vi "test Set and Get All Log File Properties.vi"(8 "error in (no error)":errorcluster, 11 "TestCase in":refnum<class "Embedded Data Logger Scripting Unit Tests.lvclass">) -> (0 "error out":errorcluster, 3 "TestCase out":refnum<class "Embedded Data Logger Scripting Unit Tests.lvclass">)   [LabVIEW 2027, in "Embedded Data Logger Scripting Unit Tests.lvclass"]
uses:
  Embedded Data Logger Scripting Unit Tests.lvclass
  C:/Program Files/National Instruments/LabVIEW 2027/vi.lib/NI/VeriStand Custom Device Testing Tools/VeriStandScriptingTestCase/VeriStandScriptingTestCase.lvclass
  Shared/Segment Files By.ctl
  <vilib>/NI/VeriStand Custom Device Testing Tools/VeriStandScriptingTestCase/VeriStandScriptingTestCase.lvclass/VeriStandScriptingTestCase.ctl
  <vilib>/NI/VeriStand Custom Device Testing Tools/VeriStandScriptingTestCase/Read Target.vi
  C:/NetCoreDLL/NationalInstruments.VeriStand.SystemDefinitionAPI.dll
  NetCoreDLL/NationalInstruments.VeriStand.SystemDefinitionAPI.dll
  Embedded Data Logger Scripting.lvlib
  Shared/Embedded Data Logger Shared.lvlib
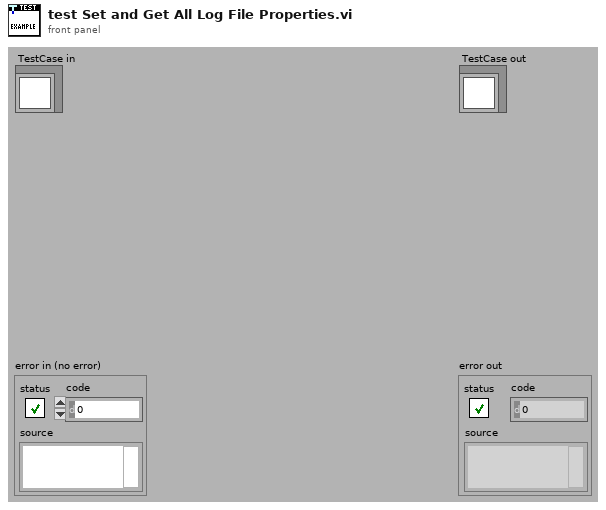
[diagram p1: front panel]
types:
  T1 = typedef "Embedded Data Logger Shared.lvlib/Segment Files By.ctl" = enum16{"Time", "Size"}
  T2 = typedef "Custom Device API.lvlib/Custom Device Item Ref.ctl" = u64
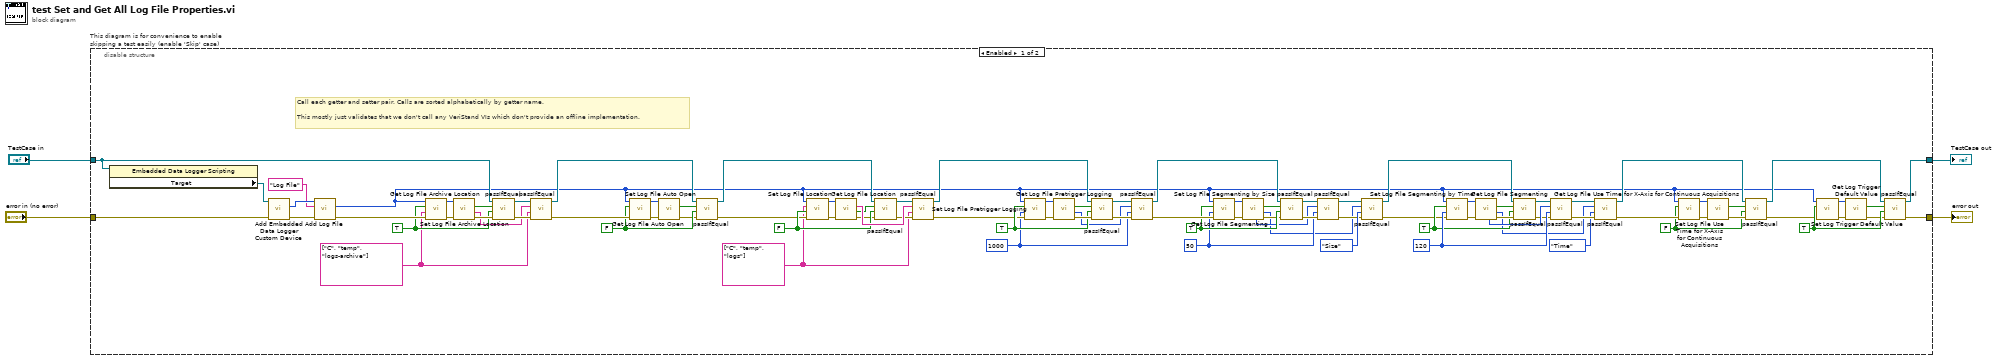
[diagram p0: block diagram]
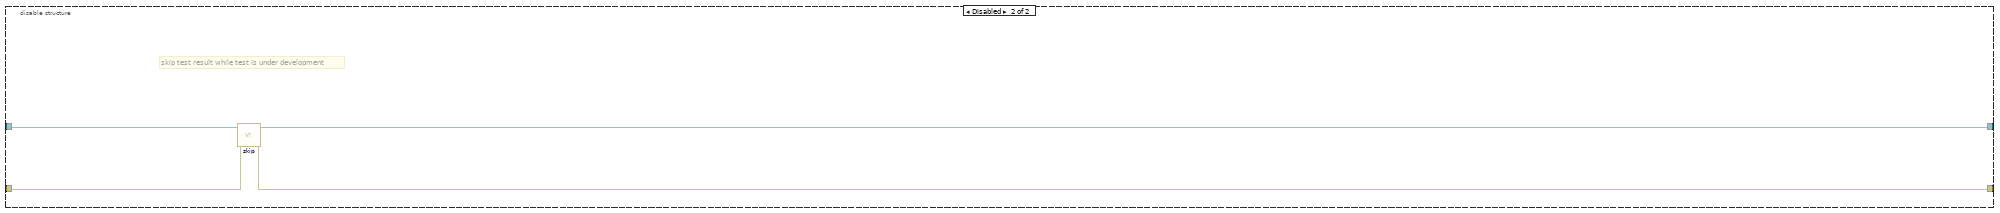
[diagram p2: hidden frame]
diagram:
  n1 = disable-structure "This diagram is for convenience to enable skipping a test easily (enable 'Skip' case)" shown="Enabled" {
    disable-tunnel: "TestCase in" -> [w86 w100]
    disable-tunnel: [w8 w98] -> w1
    disable-tunnel: [w9 w99] -> w3
    disable-tunnel: "error in (no error)" -> [w92 w97]
    frame Enabled {
      w14 = TRUE ("auto open")
      w15 = FALSE ("auto open")
      w33 = u32 120 ("file size (MB)")
      w29 = TRUE ("segment into multiple files")
      w42 = u32 50 ("file size (MB)")
      w47 = TRUE ("segment into multiple files")
      w52 = 1000 ("pretrigger samples")
      w62 = TRUE ("auto open")
      w64 = string[] ["C", "temp", "logs"] ("archive directory parts")
      w71 = FALSE ("archive closed log files")
      w76 = FALSE ("auto open")
      w83 = string[] ["C", "temp", "logs-archive"] ("archive directory parts")
      w84 = TRUE ("archive closed log files")
      # "Call each getter and setter pair. Calls are sorted alphabetically by getter name. \n\nThis mostly just validates that we don't call any VeriStand VIs which don't provide an offline implementation."
      n2 = property class="Embedded Data Logger Scripting "(reference=w86) -> ("Target"=w93:refnum<k39>)  [unwired: 1 in, 2 out]
      n3 = call "Add Embedded Data Logger Custom Device.vi"("error in"=w92, "NationalInstruments.VeriStand.SystemDefinitionAPI.Target"=w93) -> ("error out"=w95:errorcluster, "embedded data logger"=w96:T2)  [unwired: 7 in, 1 out]
      n4 = call "Add Log File.vi"("error in"=w95, "log file name"="Log File", "embedded data logger in"=w96) -> ("error out"=w89:errorcluster, "log file"=w5:T2)  [unwired: 6 in, 1 out]
      n5 = call "Set Log File Archive Location.vi"("error in (no error)"=w89, "archive directory parts"=w83, "archive closed log files"=w84, "log file in"=w5) -> ("error out"=w91:errorcluster, "log file out"=w90:T2)  [unwired: 6 in]
      n6 = call "Get Log File Archive Location.vi"("error in (no error)"=w91, "log file in"=w90) -> ("error out"=w88:errorcluster, "archive directory parts"=w82:string[], "archive closed log files"=w85:bool)  [unwired: 6 in, 1 out]
      n7 = call-dynamic "passIfEqual.vi"("error in (no error)"=w88, "y"=w84, "x"=w85, "TestCase in"=w86) -> ("error out"=w87:errorcluster, "TestCase out"=w81:refnum<class "Embedded Data Logger Scripting Unit Tests.lvclass">)  [unwired: 6 in]
      n8 = call-dynamic "passIfEqual.vi"("error in (no error)"=w87, "y"=w83, "x"=w82, "TestCase in"=w81) -> ("error out"=w80:errorcluster, "TestCase out"=w74:refnum<class "Embedded Data Logger Scripting Unit Tests.lvclass">)  [unwired: 6 in]
      n9 = call "Set Log File Auto Open.vi"("error in"=w80, "auto open"=w76, "log file in"=w5) -> ("error out"=w78:errorcluster, "log file out"=w79:T2)  [unwired: 7 in]
      n10 = call "Get Log File Auto Open.vi"("error in"=w78, "log file in"=w79) -> ("error out"=w75:errorcluster, "auto open"=w77:bool)  [unwired: 7 in, 1 out]
      n11 = call-dynamic "passIfEqual.vi"("error in (no error)"=w75, "y"=w76, "x"=w77, "TestCase in"=w74) -> ("error out"=w65:errorcluster, "TestCase out"=w57:refnum<class "Embedded Data Logger Scripting Unit Tests.lvclass">)  [unwired: 6 in]
      n12 = call "Set Log File Location.vi"("error in"=w65, "timestamp file name"=w71, "directory parts"=w64, "log file in"=w5) -> ("error out"=w66:errorcluster, "log file out"=w67:T2)  [unwired: 5 in, 1 out]
      n13 = call "Get Log File Location.vi"("error in (no error)"=w66, "log file in"=w67) -> ("error out"=w68:errorcluster, "timestamp file name"=w70:bool, "directory parts"=w72:string[])  [unwired: 4 in, 3 out]
      n14 = call-dynamic "passIfEqual.vi"("error in (no error)"=w68, "y"=w71, "x"=w70, "TestCase in"=w57) -> ("error out"=w69:errorcluster, "TestCase out"=w73:refnum<class "Embedded Data Logger Scripting Unit Tests.lvclass">)  [unwired: 6 in]
      n15 = call-dynamic "passIfEqual.vi"("error in (no error)"=w69, "y"=w64, "x"=w72, "TestCase in"=w73) -> ("error out"=w58:errorcluster, "TestCase out"=w56:refnum<class "Embedded Data Logger Scripting Unit Tests.lvclass">)  [unwired: 6 in]
      n16 = call "Set Log File Pretrigger Logging.vi"("error in"=w58, "pretrigger samples"=w52, "pretrigger logging"=w62, "log file in"=w5) -> ("error out"=w60:errorcluster, "log file out"=w59:T2)  [unwired: 6 in]
      n17 = call "Get Log File Pretrigger Logging.vi"("error in"=w60, "log file in"=w59) -> ("error out"=w63:errorcluster, "pretrigger samples"=w53:i32, "pretrigger logging"=w61:bool)  [unwired: 6 in, 1 out]
      n18 = call-dynamic "passIfEqual.vi"("error in (no error)"=w63, "y"=w62, "x"=w61, "TestCase in"=w56) -> ("error out"=w55:errorcluster, "TestCase out"=w54:refnum<class "Embedded Data Logger Scripting Unit Tests.lvclass">)  [unwired: 6 in]
      n19 = call-dynamic "passIfEqual.vi"("error in (no error)"=w55, "y"=w52, "x"=w53, "TestCase in"=w54) -> ("error out"=w51:errorcluster, "TestCase out"=w45:refnum<class "Embedded Data Logger Scripting Unit Tests.lvclass">)  [unwired: 6 in]
      n20 = call "Set Log File Segmenting by Size.vi"("error in"=w51, "file size (MB)"=w42, "segment into multiple files"=w47, "log file in"=w5) -> ("error out"=w49:errorcluster, "log file out"=w50:T2)  [unwired: 6 in]
      n21 = call "Get Log File Segmenting.vi"("error in"=w49, "log file in"=w50) -> ("error out"=w46:errorcluster, "file segmenting mode"=w24:T1, "segment into multiple files"=w48:bool, "file length (s) or size (MB)"=w41:u32)  [unwired: 5 in, 1 out]
      n22 = call-dynamic "passIfEqual.vi"("error in (no error)"=w46, "y"=w47, "x"=w48, "TestCase in"=w45) -> ("error out"=w44:errorcluster, "TestCase out"=w43:refnum<class "Embedded Data Logger Scripting Unit Tests.lvclass">)  [unwired: 6 in]
      n23 = call-dynamic "passIfEqual.vi"("error in (no error)"=w44, "y"=w42, "x"=w41, "TestCase in"=w43) -> ("error out"=w39:errorcluster, "TestCase out"=w38:refnum<class "Embedded Data Logger Scripting Unit Tests.lvclass">)  [unwired: 6 in]
      n24 = call-dynamic "passIfEqual.vi"("error in (no error)"=w39, "y"=Segment_Files_By."Size" ("file segmenting mode"), "x"=w24, "TestCase in"=w38) -> ("error out"=w25:errorcluster, "TestCase out"=w22:refnum<class "Embedded Data Logger Scripting Unit Tests.lvclass">)  [unwired: 6 in]
      n25 = call "Set Log File Segmenting by Time.vi"("error in"=w25, "file length (s)"=w33, "segment into multiple files"=w29, "log file in"=w5) -> ("error out"=w27:errorcluster, "log file out"=w26:T2)  [unwired: 6 in]
      n26 = call "Get Log File Segmenting.vi"("error in"=w27, "log file in"=w26) -> ("error out"=w30:errorcluster, "file segmenting mode"=w23:T1, "segment into multiple files"=w28:bool, "file length (s) or size (MB)"=w34:u32)  [unwired: 5 in, 1 out]
      n27 = call-dynamic "passIfEqual.vi"("error in (no error)"=w30, "y"=w29, "x"=w28, "TestCase in"=w22) -> ("error out"=w31:errorcluster, "TestCase out"=w32:refnum<class "Embedded Data Logger Scripting Unit Tests.lvclass">)  [unwired: 6 in]
      n28 = call-dynamic "passIfEqual.vi"("error in (no error)"=w31, "y"=w33, "x"=w34, "TestCase in"=w32) -> ("error out"=w36:errorcluster, "TestCase out"=w37:refnum<class "Embedded Data Logger Scripting Unit Tests.lvclass">)  [unwired: 6 in]
      n29 = call-dynamic "passIfEqual.vi"("error in (no error)"=w36, "y"=Segment_Files_By."Time" ("file segmenting mode"), "x"=w23, "TestCase in"=w37) -> ("error out"=w16:errorcluster, "TestCase out"=w19:refnum<class "Embedded Data Logger Scripting Unit Tests.lvclass">)  [unwired: 6 in]
      n30 = call "Set Log File Use Time for X-Axis for Continuous Acquisitions.vi"("error in"=w16, "use time for x-axis for continuous acquisitions"=w15, "log file in"=w5) -> ("error out"=w17:errorcluster, "log file out"=w20:T2)  [unwired: 7 in]
      n31 = call "Get Log File Use Time for X-Axis for Continuous Acquisitions.vi"("error in"=w17, "log file in"=w20) -> ("error out"=w18:errorcluster, "use time for x-axis for continuous acquisitions"=w21:bool)  [unwired: 7 in, 1 out]
      n32 = call-dynamic "passIfEqual.vi"("error in (no error)"=w18, "y"=w15, "x"=w21, "TestCase in"=w19) -> ("error out"=w6:errorcluster, "TestCase out"=w7:refnum<class "Embedded Data Logger Scripting Unit Tests.lvclass">)  [unwired: 6 in]
      n33 = call "Set Log Trigger Default Value.vi"("error in"=w6, "log trigger default value"=w14, "log file in"=w5) -> ("error out"=w13:errorcluster, "log file out"=w11:T2)  [unwired: 7 in]
      n34 = call "Get Log Trigger Default Value.vi"("error in"=w13, "log file in"=w11) -> ("error out"=w12:errorcluster, "log trigger default value"=w10:bool)  [unwired: 7 in, 1 out]
      n35 = call-dynamic "passIfEqual.vi"("error in (no error)"=w12, "y"=w14, "x"=w10, "TestCase in"=w7) -> ("error out"=w9:errorcluster, "TestCase out"=w8:refnum<class "Embedded Data Logger Scripting Unit Tests.lvclass">)  [unwired: 6 in]
    }
    frame Disabled {
      # "skip test result while test is under development"
      n36 = call <vilib>:"skip.vi"("error in (no error)"=w97, "TestCase in"=w100) -> ("error out"=w99:errorcluster, "TestCase out"=w98:refnum<class "Embedded Data Logger Scripting Unit Tests.lvclass">)  [unwired: 8 in]
    }
  }
  "error out" <- w3
  "TestCase out" <- w1
